vi "ReadValue.vi"(0 "reference in":refnum<class "Switch_MotorP5.lvclass">, 2 "Name":string, 5 "error in (no error)":errorcluster) -> (14 "reference in":refnum<class "Switch_MotorP5.lvclass">, 16 "Value":dbl, 19 "error out":errorcluster)   [LabVIEW 2022 SP3, in "Switch_MotorP5.lvlib" / "Switch_MotorP5.lvclass"]
uses:
  Switch_MotorP5.lvclass
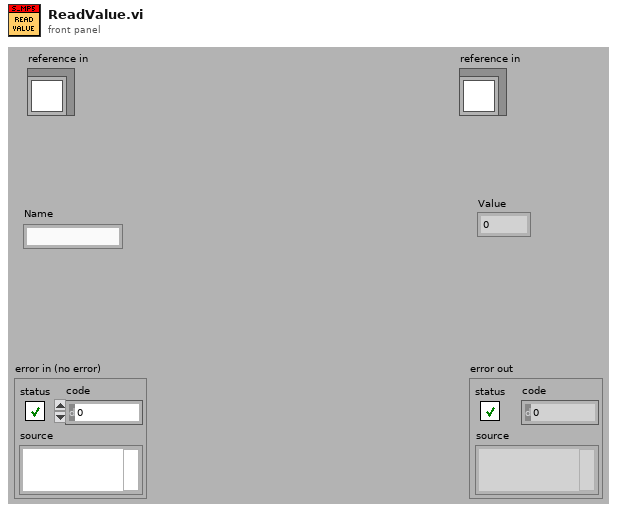
[diagram p1: front panel]
types:
  T1 = typedef "Switch_MotorP5.lvlib/Switch_MotorP5.lvclass/ObjectAttributes.ctl" = cluster{"Config":T2, "VISA":refnum<visa-resource-name>, "RPM":i32, "States":bool[], "UpdateEvent":refnum<user-event>, "Motor":enum32{"M1", "M2", "M3", "M4", "M5", "M6", "M7", "M8"}}
  T2 = typedef "Switch_MotorP5.lvlib/Switch_MotorP5.lvclass/Config.ctl" = cluster{"COM":refnum<visa-resource-name>, "SwitchMap":cluster{"Name":string, "Description":string, "Group":string, "IsGroup":bool, "Motor":enum32{"M1", "M2", "M3", "M4", "M5", "M6", "M7", "M8", "NA"}}[], "Sim":bool}
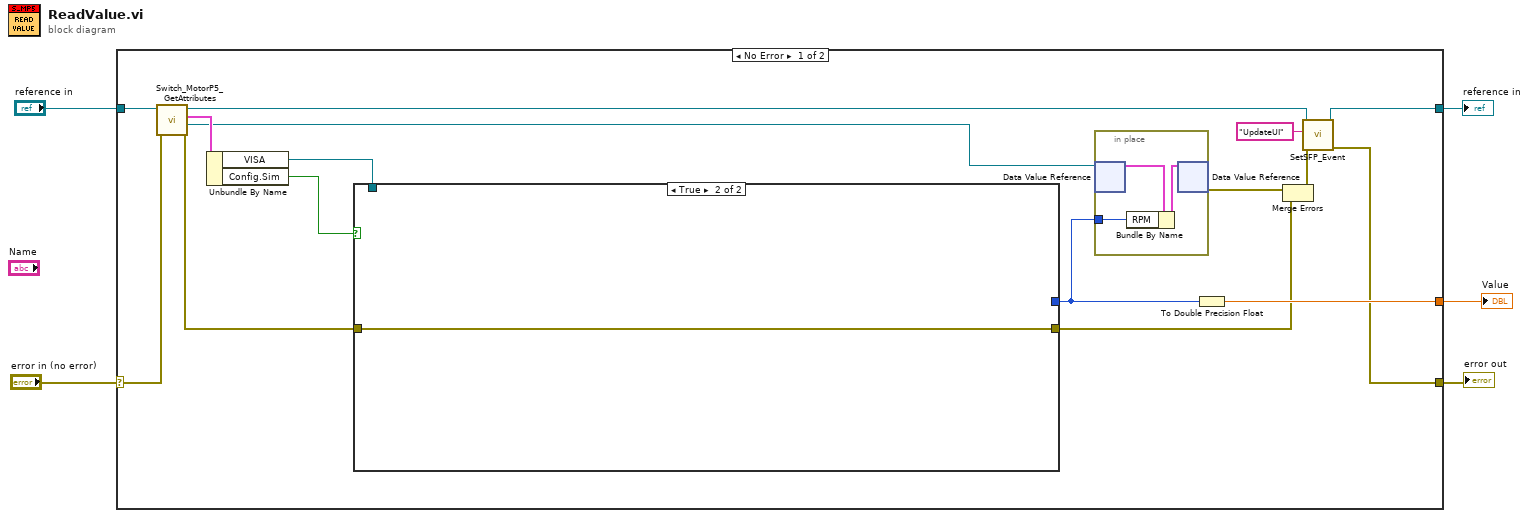
[diagram p0: block diagram]
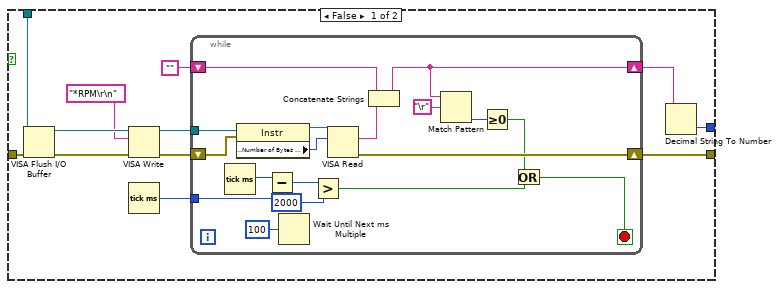
[diagram p2: hidden frame]
diagram:
  n1 = case shown="No Error" "error in (no error)" {
    selector: "error in (no error)" -> [w21 w57]
    tunnel: [w9 w57] -> w4
    tunnel: [w12 w56] -> w2
    tunnel: "reference in" -> [w19 w56]
    tunnel: [w16 _] -> w1
    frame No Error {
      n2 = call "Switch_MotorP5_GetAttributes.vi"("error in (no error)"=w21, "reference in"=w19) -> ("error out"=w17:errorcluster, "DataRef"=w11:refnum<data-value>, "Data"=w20:T1, "reference out"=w13:refnum<class "Switch_MotorP5.lvclass">)  [unwired: 6 in]
      n3 = Unbundle By Name(w20) -> ("VISA"=w18:refnum<visa-resource-name>, "Config.Sim"=w6:bool)
      n4 = case shown="True" w6 {
        tunnel: w18 -> [w33 _]
        tunnel: w17 -> [w29 w52]
        tunnel: [w28 w52] -> w10
        tunnel: [w27 _] -> w7
        frame False {
          n5 = VISA Flush I/O Buffer(VISA resource name=w33, error in (no error)=w29) -> (VISA resource name out=w31:refnum<visa-resource-name>, error out=w32:errorcluster)  [unwired: 1 in]
          n6 = VISA Write(VISA resource name=w31, write buffer="*RPM\r\n", error in (no error)=w32) -> (VISA resource name out=w26:refnum<visa-resource-name>, error out=w25:errorcluster)  [unwired: 1 out]
          n7 = Tick Count (ms)() -> (millisecond timer value=w24:u32)
          n8 = while {
            tunnel: w26 -> [w50]
            shift-right: [w51] -> w28
            shift-left: w25 -> [w48]
            tunnel: w24 -> [w44]
            shift-right: [w39] -> w22
            shift-left: "" -> [w40]
            stop <- w34 stop-if-true
            n9 = Tick Count (ms)() -> (millisecond timer value=w45:u32)
            n10 = property class="Instr"(reference=w50, error in=w48) -> (reference out=w47:refnum<visa-resource-name>, "Serial Settings:Number of Bytes at Serial Port"=w49:u32)  [unwired: 1 out]
            n11 = Subtract(x=w45, y=w44) -> (x-y=w43:u32)
            n12 = Wait Until Next ms Multiple(millisecond multiple=u32 100) -> ()  [unwired: 1 out]
            n13 = Greater?(x=w43, y=u32 2000) -> (0:w35:bool)
            n14 = VISA Read(VISA resource name=w47, byte count=w49) -> (read buffer=w41:string, error out=w51:errorcluster)  [unwired: 1 in, 2 out]
            n15 = Concatenate Strings(w40, w41) -> (w39:string)
            n16 = Match Pattern(string=w39, regular expression="\r") -> (offset past match=w37:i32)  [unwired: 1 in, 3 out]
            n17 = Greater Or Equal To 0?(x=w37) -> (x >= 0?=w36:bool)
            n18 = Or(x=w36, y=w35) -> (x .or. y?=w34:bool)
          }
          n19 = Decimal String To Number(string=w22) -> (number=w27:i32)  [unwired: 2 in, 1 out]
        }
        frame True {
        }
      }
      n20 = in-place {
        in-place-border: w7 -> [w53]
        n21 = in-place-dvr #1(w11) -> (w55:T1)  [unwired: 1 out]
        n22 = Bundle By Name(cluster=w55, "RPM"=w53) -> (w54:T1)
        n23 = in-place-dvr #1(w54) -> (w8:errorcluster)  [unwired: 1 out]
      }
      n24 = To Double Precision Float(number=w7) -> (double precision float=w16:dbl)
      n25 = Merge Errors(w8, w10) -> (w15:errorcluster)
      n26 = call-dynamic "SetSFP_Event.vi"("error in (no error)"=w15, "msg"="UpdateUI", "reference in"=w13) -> ("error out"=w9:errorcluster, "reference out"=w12:refnum<class "Switch_MotorP5.lvclass">)  [unwired: 7 in]
    }
    frame Error {
    }
  }
  "error out" <- w4
  "reference in" <- w2
  "Value" <- w1
